vi "QuitProg.vi"() -> ()   [LabVIEW 2011]
panel:
  out "QuitProg.":bool
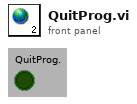
[diagram p1: front panel]
diagram:
